vi "Seven_Segment.vi"() -> ()   [LabVIEW 2024]
panel:
  in  "Numeric":i32
  out "Boolean 4":bool
  out "Boolean 7":bool
  out "Boolean 3":bool
  out "Boolean 5":bool
  out "Boolean 6":bool
  out "Boolean 2":bool
  out "Boolean 1":bool
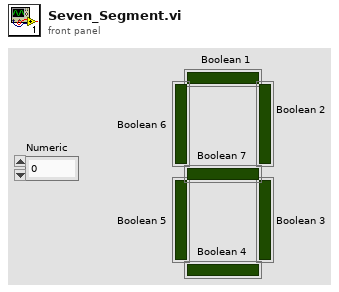
[diagram p1: front panel]
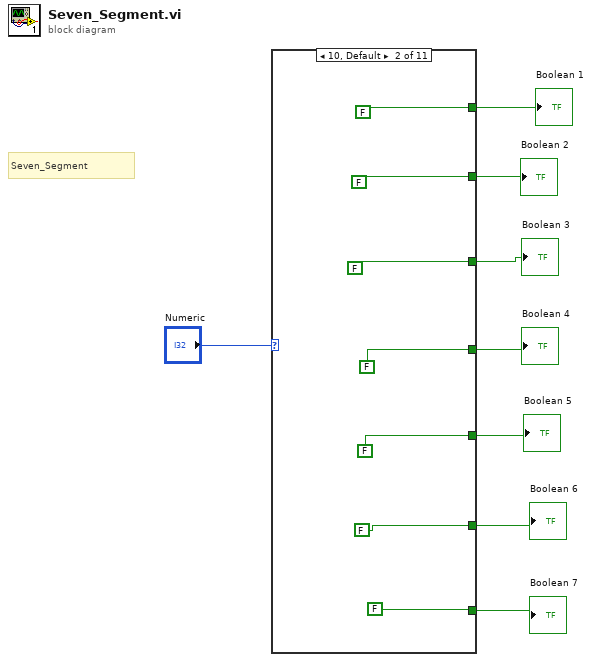
[diagram p0: block diagram]
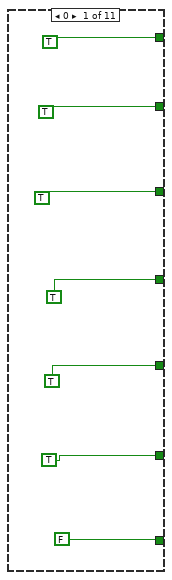
[diagram p2: hidden frame]
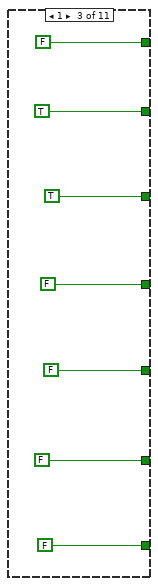
[diagram p3: hidden frame]
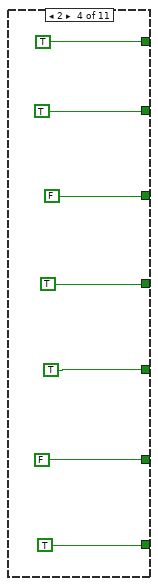
[diagram p4: hidden frame]
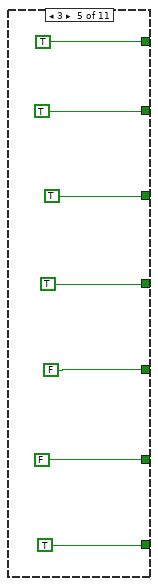
[diagram p5: hidden frame]
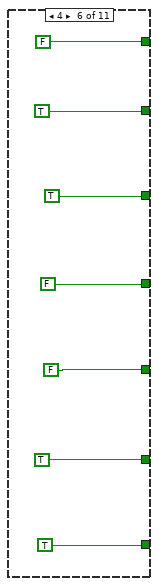
[diagram p6: hidden frame]
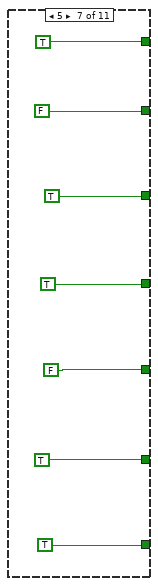
[diagram p7: hidden frame]
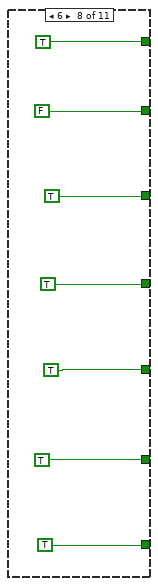
[diagram p8: hidden frame]
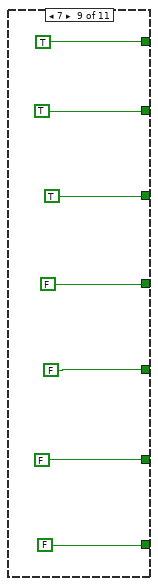
[diagram p9: hidden frame]
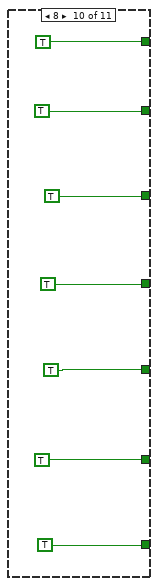
[diagram p10: hidden frame]
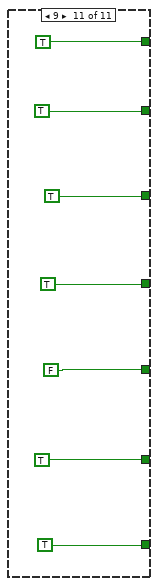
[diagram p11: hidden frame]
diagram:
  # "Seven_Segment"
  n1 = case shown="10, Default" "Numeric" {
    tunnel: [TRUE FALSE FALSE TRUE TRUE FALSE TRUE TRUE TRUE TRUE TRUE] -> w8
    tunnel: [TRUE FALSE TRUE TRUE TRUE TRUE FALSE FALSE TRUE TRUE TRUE] -> w7
    tunnel: [TRUE FALSE TRUE FALSE TRUE TRUE TRUE TRUE TRUE TRUE TRUE] -> w6
    tunnel: [TRUE FALSE FALSE TRUE TRUE FALSE TRUE TRUE FALSE TRUE TRUE] -> w5
    tunnel: [TRUE FALSE FALSE TRUE FALSE FALSE FALSE TRUE FALSE TRUE FALSE] -> w4
    tunnel: [TRUE FALSE FALSE FALSE FALSE TRUE TRUE TRUE FALSE TRUE TRUE] -> w3
    tunnel: [FALSE FALSE FALSE TRUE TRUE TRUE TRUE TRUE FALSE TRUE TRUE] -> w2
    frame 0 {
    }
    frame 10, Default {
    }
    frame 1 {
    }
    frame 2 {
    }
    frame 3 {
    }
    frame 4 {
    }
    frame 5 {
    }
    frame 6 {
    }
    frame 7 {
    }
    frame 8 {
    }
    frame 9 {
    }
  }
  "Boolean 1" <- w8
  "Boolean 2" <- w7
  "Boolean 6" <- w3
  "Boolean 5" <- w4
  "Boolean 3" <- w6
  "Boolean 7" <- w2
  "Boolean 4" <- w5
